vi "collectPelvicBounds.vi"() -> (0 "yzgraph array":cluster{dbl[], dbl[]}[](array[cluster]), 3 "xzgraph":cluster{dbl[], dbl[]}[](array[cluster]))   [LabVIEW 2024]
panel:
  out "yz Currentpt":cluster{dbl[], dbl[]}
  out "xz Currentpt":cluster{dbl[], dbl[]}
  out "xzCenterpel":cluster{dbl[], dbl[]}
  out "yzboundsCluster":cluster{dbl[], dbl[]}
  out "yzCenterPel":cluster{dbl[], dbl[]}
  out "xzboundsCluster":cluster{dbl[], dbl[]}
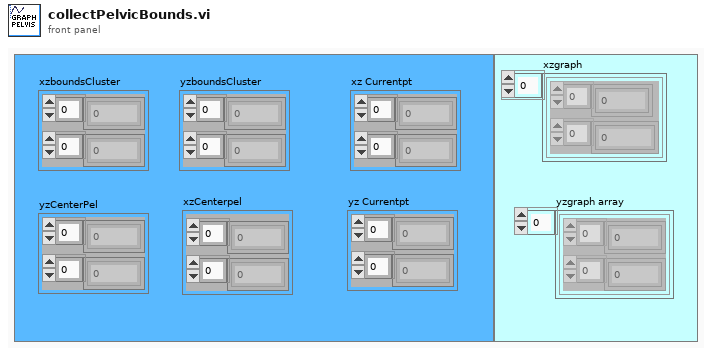
[diagram p1: front panel]
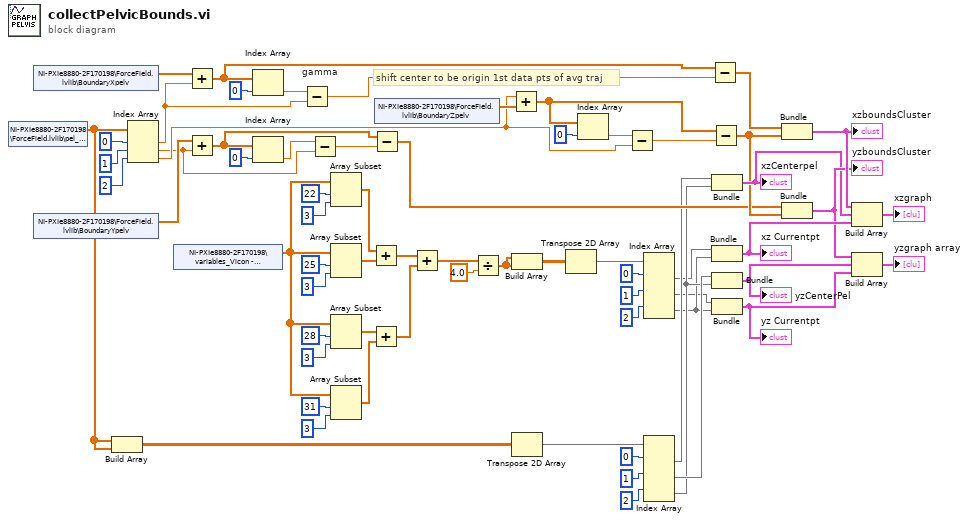
[diagram p0: block diagram]
diagram:
  # "shift center to be origin 1st data pts of avg traj"
  n1 = shared-variable "NI-PXIe8880-2F170198\\ForceField.lvlib\\pel_cn"() -> (w7:dbl[])  [unwired: 1 in, 1 out]
  n2 = shared-variable "NI-PXIe8880-2F170198\\ForceField.lvlib\\BoundaryXpelv"() -> (w66:dbl[])  [unwired: 1 in, 1 out]
  n3 = shared-variable "NI-PXIe8880-2F170198\\ForceField.lvlib\\BoundaryYpelv"() -> (w60:dbl[])  [unwired: 1 in, 1 out]
  n4 = Build Array(w7, w7) -> (w64:dbl[][])
  n5 = Index Array(array=w7, index #1=0 ("index"), index #2=1 ("index"), index #3=2 ("index")) -> (element #1=w23:dbl, element #2=w12:dbl, element #3=w19:dbl)
  n6 = shared-variable "NI-PXIe8880-2F170198\\variables_Vicon - networkPublished.lvlib\\viconData_2"() -> (w44:dbl[])  [unwired: 1 in, 1 out]
  n7 = Add(x=w66, y=w23) -> (x+y=w21:dbl[])
  n8 = Add(x=w60, y=w12) -> (x+y=w14:dbl[])
  n9 = Index Array(array=w21, index=0) -> (element=w22:dbl)
  n10 = Index Array(array=w14, index=0) -> (element=w11:dbl)
  n11 = Subtract "gamma"(x=w22, y=w23) -> (x-y=w20:dbl)
  n12 = Subtract(x=w11, y=w12) -> (x-y=w13:dbl)
  n13 = Array Subset(array=w44, index=22, length=3) -> (w52:dbl[])
  n14 = Array Subset(array=w44, index=25, length=3) -> (w53:dbl[])
  n15 = Array Subset(array=w44, index=28, length=3) -> (w54:dbl[])
  n16 = Array Subset(array=w44, index=31, length=3) -> (w55:dbl[])
  n17 = Add(x=w52, y=w53) -> (x+y=w57:dbl[])
  n18 = Add(x=w54, y=w55) -> (x+y=w56:dbl[])
  n19 = Subtract(x=w14, y=w13) -> (x-y=w9:dbl[])
  n20 = shared-variable "NI-PXIe8880-2F170198\\ForceField.lvlib\\BoundaryZpelv"() -> (w65:dbl[])  [unwired: 1 in, 1 out]
  n21 = Add(x=w57, y=w56) -> (x+y=w43:dbl[])
  n22 = Divide(x=w43, y=4.0) -> (x/y=w39:dbl[])
  n23 = Add(x=w19, y=w65) -> (x+y=w8:dbl[])
  n24 = Build Array(w39, w39) -> (w38:dbl[][])
  n25 = Transpose 2D Array(2D array=w64) -> (transposed array=w62:dbl[][])
  n26 = Transpose 2D Array(2D array=w38) -> (transposed array=w37:dbl[][])
  n27 = Index Array(array=w8, index=0) -> (element=w18:dbl)
  n28 = Subtract(x=w18, y=w19) -> (x-y=w17:dbl)
  n29 = Index Array(array=w37, index (row) #1=0 ("index (row)"), index (row) #2=1 ("index (row)"), index (row) #3=2 ("index (row)")) -> (element #1=w1:dbl[], element #2=w2:dbl[], element #3=w3:dbl[])  [unwired: 3 in]
  n30 = Index Array(array=w62, index (row) #1=0 ("index (row)"), index (row) #2=1 ("index (row)"), index (row) #3=2 ("index (row)")) -> (element #1=w6:dbl[], element #2=w5:dbl[], element #3=w4:dbl[])  [unwired: 3 in]
  n31 = Subtract(x=w21, y=w20) -> (x-y=w10:dbl[])
  n32 = Subtract(x=w8, y=w17) -> (x-y=w16:dbl[])
  n33 = Bundle(w6, w4) -> (w30:cluster{dbl[], dbl[]})  [unwired: 1 in]
  "xzCenterpel" <- w30
  n34 = Bundle(w1, w3) -> (w32:cluster{dbl[], dbl[]})  [unwired: 1 in]
  "xz Currentpt" <- w32
  n35 = Bundle(w5, w4) -> (w26:cluster{dbl[], dbl[]})  [unwired: 1 in]
  "yzCenterPel" <- w26
  n36 = Bundle(w2, w3) -> (w29:cluster{dbl[], dbl[]})  [unwired: 1 in]
  "yz Currentpt" <- w29
  n37 = Bundle(w10, w16) -> (w33:cluster{dbl[], dbl[]})  [unwired: 1 in]
  "xzboundsCluster" <- w33
  n38 = Bundle(w9, w16) -> (w31:cluster{dbl[], dbl[]})  [unwired: 1 in]
  "yzboundsCluster" <- w31
  n39 = Build Array(w33, w30, w32) -> (→"xzgraph":cluster{dbl[], dbl[]}[])
  n40 = Build Array(w31, w26, w29) -> (→"yzgraph array":cluster{dbl[], dbl[]}[])
